vi "RichToFlatnixnet_grpc_StatusToStringRequest.vi"(5 "OutputClusterType":T1, 11 "InputCluster":T2) -> (3 "OutputCluster":T1)   [LabVIEW 2025, in "grpc-xnet_client.lvlib"]
uses:
  grpc-xnet_client.lvlib
  nixnet_grpc_StatusToStringRequest.ctl
  nixnet_grpc_StatusToStringRequest_Flat.ctl
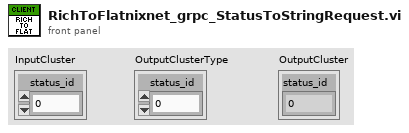
[diagram p1: front panel]
types:
  T1 = typedef "grpc-xnet_client.lvlib/nixnet_grpc_StatusToStringRequest_Flat.ctl" = cluster{"status_id":i32}
  T2 = typedef "grpc-xnet_client.lvlib/nixnet_grpc_StatusToStringRequest.ctl" = cluster{"status_id":i32}
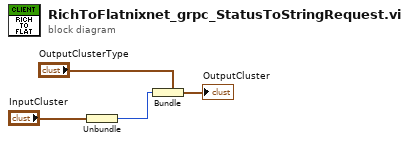
[diagram p0: block diagram]
diagram:
  n1 = Unbundle "Unbundle"("InputCluster") -> ("status_id"=w1:i32)
  n2 = Bundle "Bundle"(cluster="OutputClusterType", "status_id"=w1) -> (→"OutputCluster":T1)
